vi "increase_revision.vi"(8 "error in (no error)":errorcluster, 11 "GenericPlugin in":refnum<class "GenericComponent.lvclass">) -> (0 "error out":errorcluster, 2 "new LSID":T1, 3 "GenericPlugin out":refnum<class "GenericComponent.lvclass">)   [LabVIEW 2010, in "GenericComponent.lvclass"]
uses:
  GenericComponent.lvclass
  clusters/LSID_cluster.ctl
  GenericComponent.lvclass/GenericComponent.ctl
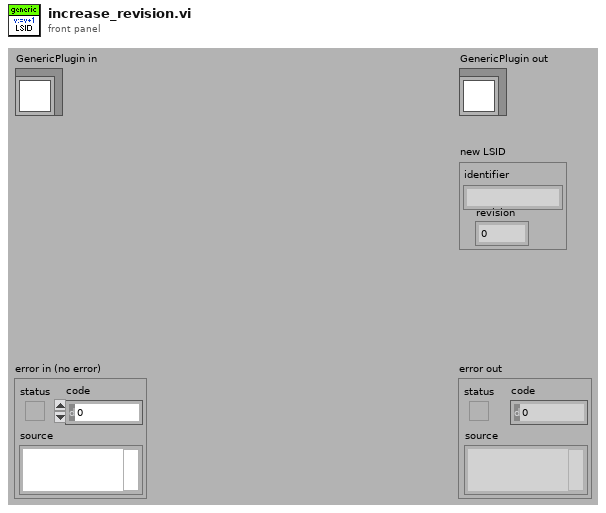
[diagram p1: front panel]
types:
  T1 = typedef "LSID_cluster.ctl" = cluster{"identifier":string, "revision":i32}
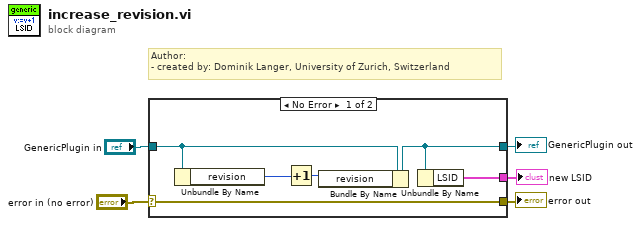
[diagram p0: block diagram]
diagram:
  # "Author: \n- created by: Dominik Langer, University of Zurich, Switzerland"
  n1 = case shown="No Error" "error in (no error)" {
    selector: "error in (no error)" -> [w11 w13]
    tunnel: [w11 w13] -> w4
    tunnel: [w7 w12] -> w2
    tunnel: "GenericPlugin in" -> [w10 w12]
    tunnel: [w6 _] -> w1
    frame No Error {
      n2 = Unbundle By Name(w10) -> ("revision"=w9:i32)
      n3 = Increment(x=w9) -> (x+1=w8:i32)
      n4 = Bundle By Name(cluster=w10, "revision"=w8) -> (w7:refnum<class "GenericComponent.lvclass">)
      n5 = Unbundle By Name(w7) -> ("LSID"=w6:T1)
    }
    frame Error {
    }
  }
  "error out" <- w4
  "GenericPlugin out" <- w2
  "new LSID" <- w1
